vi "create_instance_by_specification.vi"(6 "be tolerant against empty specification?":bool, 7 "call constructor?":bool, 8 "error in (no error)":errorcluster, 11 "component specification":T1) -> (0 "error out":errorcluster, 2 "empty specification!":bool, 3 "GenericPlugin out":refnum<class "GenericComponent.lvclass">)   [LabVIEW 2010, in "GenericComponent.lvclass"]
uses:
  GenericComponent.lvclass
  clusters/plugin_specification.ctl
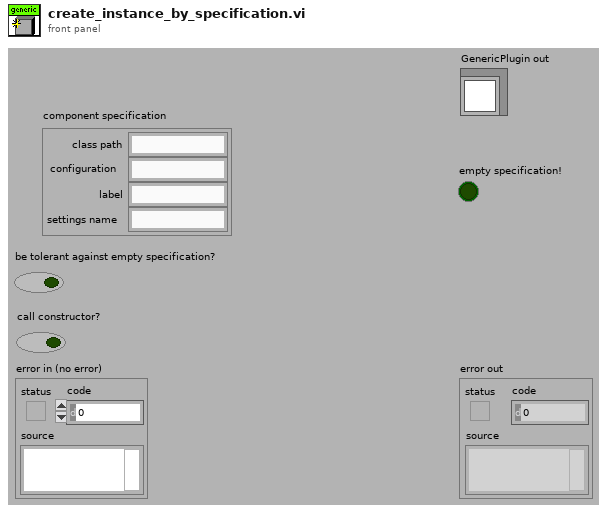
[diagram p1: front panel]
types:
  T1 = typedef "plugin_specification.ctl" = cluster{"class path":string, "configuration":string, "label":string, "settings name":string}
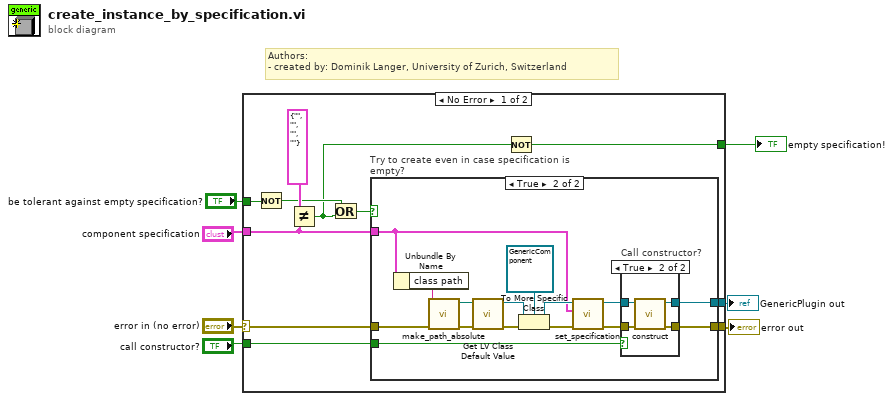
[diagram p0: block diagram]
diagram:
  # "Authors: \n- created by: Dominik Langer, University of Zurich, Switzerland"
  n1 = case shown="No Error" "error in (no error)" {
    selector: "error in (no error)" -> [w18 w41]
    tunnel: [w17 w41] -> w6
    tunnel: [w16 _] -> w5
    tunnel: "component specification" -> [w15 _]
    tunnel: "be tolerant against empty specification?" -> [w13 _]
    tunnel: [w9 _] -> w2
    tunnel: "call constructor?" -> [w8 _]
    frame No Error {
      n2 = Not(x=w13) -> (.not. x?=w12:bool)
      n3 = Not Equal?(x=T1 {"class path"="", "configuration"="", "label"="", "settings name"=""} ("component specification"), y=w15) -> (x != y?=w10:bool)
      n4 = Or(x=w12, y=w10) -> (x .or. y?=w11:bool)
      n5 = case "Try to create even in case specification is empty?" shown="True" w11 {
        tunnel: w15 -> [_ w20]
        tunnel: w18 -> [w19 w28]
        tunnel: [w19 w31] -> w17
        tunnel: [_ w30] -> w16
        tunnel: w8 -> [_ w29]
        frame False {
        }
        frame True {
          n6 = Unbundle By Name(w20) -> ("class path"=w26:string)
          n7 = call "make_path_absolute.vi"("error in (no error)"=w28, "relative path"=w26) -> ("error out"=w27:errorcluster, "absolute path"=w25:path)  [unwired: 8 in]
          n8 = call <vilib>:"Get LV Class Default Value.vi"("error in (no error)"=w27, "class path"=w25) -> ("error out"=w34:errorcluster, "object"=w33:refnum<class>)  [unwired: 8 in]
          n9 = To More Specific Class(target class=refnum<class "GenericComponent.lvclass"> refnum ("GenericPlugin.lvclass"), reference=w33, error in=w34) -> (specific class reference=w22:refnum<class "GenericComponent.lvclass">, error out=w24:errorcluster)
          n10 = call-dynamic "set_specification.vi"("error in (no error)"=w24, "component specification"=w20, "GenericPlugin in"=w22) -> ("error out"=w23:errorcluster, "GenericPlugin out"=w21:refnum<class "GenericComponent.lvclass">)  [unwired: 7 in]
          n11 = case "Call constructor?" shown="True" w29 {
            tunnel: w23 -> [w35 w40]
            tunnel: [w35 w39] -> w31
            tunnel: w21 -> [w36 w37]
            tunnel: [w36 w38] -> w30
            frame False {
            }
            frame True {
              n12 = call-dynamic "construct.vi"("error in (no error)"=w40, "GenericPlugin in"=w37) -> ("error out"=w39:errorcluster, "GenericPlugin out"=w38:refnum<class "GenericComponent.lvclass">)  [unwired: 8 in]
            }
          }
        }
      }
      n13 = Not(x=w10) -> (.not. x?=w9:bool)
    }
    frame Error {
    }
  }
  "error out" <- w6
  "GenericPlugin out" <- w5
  "empty specification!" <- w2
